vi "cRIO_4DoF_Delta_forward_kinematics.vi"(9 "theta3":dbl, 10 "theta2":dbl, 11 "theta1":dbl) -> (1 "YD":cdb, 2 "ZD":cdb, 3 "discriminant (>0)":dbl, 4 "XD":cdb)   [LabVIEW 2019]
uses:
  Global 1.vi
  <vilib>/imath/engines/lvmath2/RunTimeEngine/Managers/WorkSpace/UID Generator.vi
  <vilib>/imath/engines/lvmath2/RunTimeEngine/RunTimeType/NIMS_RunTimeType_From StrictType (excl LVString).vi
  <instcachedir>/0/NIMS_RunTimeType_From StrictType (excl LVString)_D8AFBA86A94845AAA577C895450664BD.lvgen/NIMS_RunTimeType_From StrictType (excl LVString)_D8AFBA86A94845AAA577C895450664BD_000.vi
  <vilib>/imath/engines/lvmath2/RunTimeEngine/LocalVariableDefStatement/MC_LocalVariableDefStatement_Display.vi
  <vilib>/imath/engines/lvmath2/RunTimeEngine/Managers/SymbolTable/Clear UID.vi
  <vilib>/imath/engines/lvmath2/RunTimeEngine/NodeEndStatement/NIMS_NodeEndStatement_Output.vi
  <instcachedir>/0/NIMS_NodeEndStatement_Output_53EC0D466D134D7ABD903AC30B43404B.lvgen/NIMS_NodeEndStatement_Output_53EC0D466D134D7ABD903AC30B43404B_001.vi
  <instcachedir>/0/NIMS_NodeEndStatement_Output_53EC0D466D134D7ABD903AC30B43404B.lvgen/NIMS_NodeEndStatement_Output_53EC0D466D134D7ABD903AC30B43404B_009.vi
  <vilib>/imath/engines/lvmath2/RunTimeEngine/ErrorHandling/NIMS_Finalize Error.vi
  <vilib>/imath/engines/lvmath2/RunTimeEngine/Managers/SymbolTable/NIMS_WorkSpace.lvlib
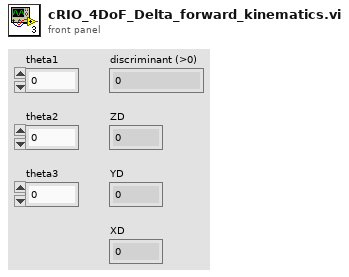
[diagram p1: front panel]
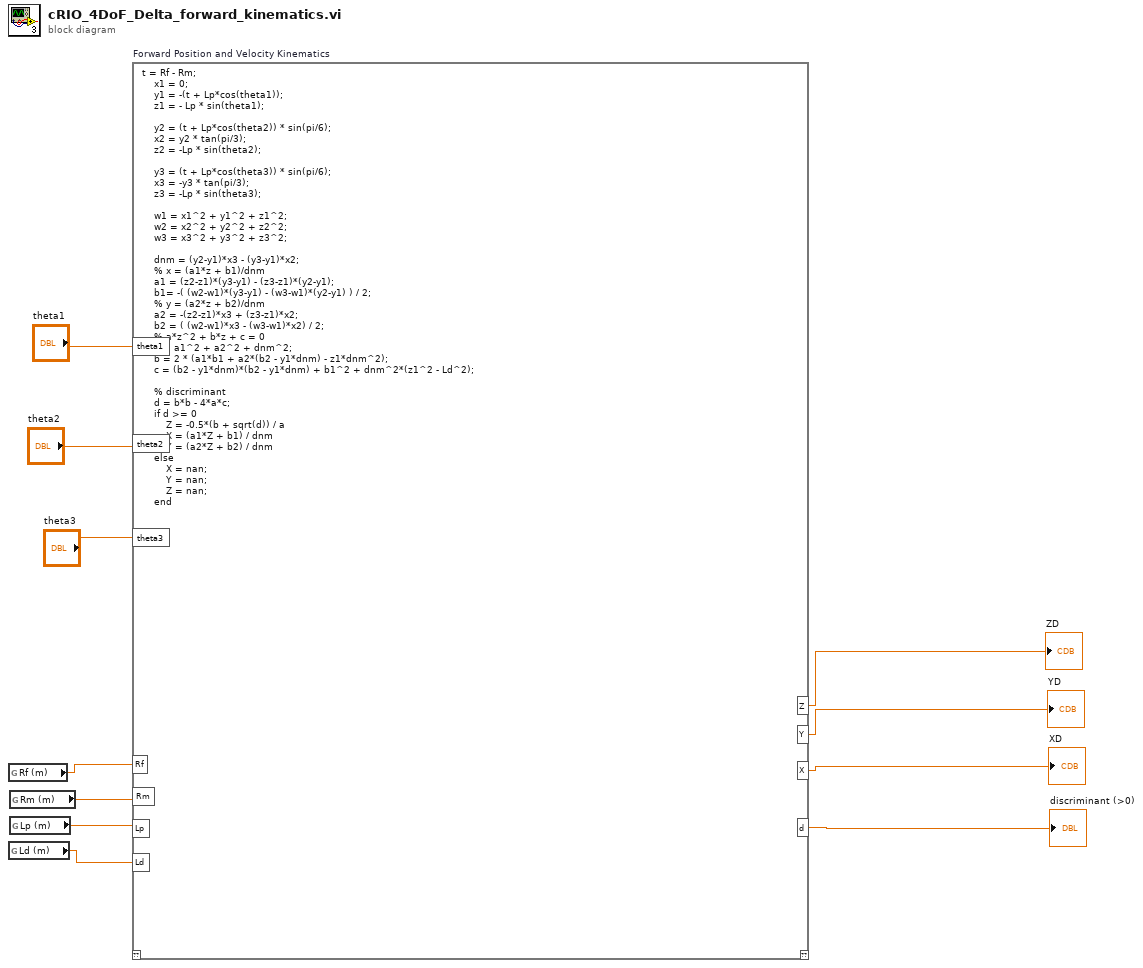
[diagram p0: block diagram]
diagram:
  n1 = global read "Global 1.vi" "Rf (m)"() -> (w4:dbl)
  n2 = global read "Global 1.vi" "Ld (m)"() -> (w1:dbl)
  n3 = global read "Global 1.vi" "Rm (m)"() -> (w3:dbl)
  n4 = global read "Global 1.vi" "Lp (m)"() -> (w2:dbl)
  n5 = mathscript code="t = Rf - Rm;\n    x1 = 0;\n    y1 = -(t + Lp*cos(theta1));\n    z1 = - Lp * sin(theta1);\n    \n    y2 = (t + Lp*cos(theta2)) * sin(pi/6);\n    x2 = y2 * tan(pi/3);\n    z2 = -Lp * sin(theta2);\n    \n    y3 = (t + Lp*cos(theta3)) * sin(pi/6);\n    x3 = -y3 * tan(pi/3);\n    z3 = -Lp * sin(theta3);\n    \n    w1 = x1^2 + y1^2 + z1^2;\n    w2 = x2^2 + y2^2 + z2^2;\n    w3 = x3^2 + y3^2 + z3^2;\n\n    dnm = (y2-y1)*x3 - (y3-y1)*x2;\n    % x = (a1*z + b1)/dnm\n    a1 = (z2-z1)*(y3-y1) - (z3-z1)*(y2-y1);\n    b1= -( (w2-w1)*(y3-y1) - (w3-w1)*(y2-y1) ) / 2;\n    % y = (a2*z + b2)/dnm\n    a2 = -(z2-z1)*x3 + (z3-z1)*x2;\n    b2 = ( (w2-w1)*x3 - (w3-w1)*x2) / 2;\n    % a*z^2 + b*z + c = 0\n    a = a1^2 + a2^2 + dnm^2;\n    b = 2 * (a1*b1 + a2*(b2 - y1*dnm) - z1*dnm^2);\n    c = (b2 - y1*dnm)*(b2 - y1*dnm) + b1^2 + dnm^2*(z1^2 - Ld^2);\n\n    % discriminant\n    d = b*b - 4*a*c;\n    if d >= 0\n        Z = -0.5*(b + sqrt(d)) / a\n        X = (a1*Z + b1) / dnm\n        Y = (a2*Z + b2) / dnm\n    else\n        X = nan;\n        Y = nan;\n        Z = nan;\n    end" "Forward Position and Velocity Kinematics"("Rf"=w4, "Rm"=w3, "Lp"=w2, "Ld"=w1, "theta1"="theta1", "theta2"="theta2", "theta3"="theta3") -> ("X"=→"XD":cdb, "Y"=→"YD":cdb, "Z"=→"ZD":cdb, "d"=→"discriminant (>0)":dbl)  [unwired: 1 in, 1 out]
